vi "Get Status of Monkeys.vi"(8 "error in (no error)":errorcluster, 11 "Tamer in":refnum<class "Tamer.lvclass">) -> (0 "error out":errorcluster, 2 "Anything running?":bool, 3 "Tamer out":refnum<class "Tamer.lvclass">)   [LabVIEW 2020, in "Tamer.lvlib" / "Tamer.lvclass"]
doc: "Check if any Monkey is running"
uses:
  Tamer.lvclass
  Tamer.lvclass/Tamer.ctl
  Ancestor/Ancestor/Ancestor.lvclass/Ancestor.ctl
  Support VIs/Generate Error.vi
  FGV/Error Memory/Get Error Description.vi
  Support VIs/Get PC name.vi
  Ancestor/Ancestor/Read ID.vi
  Support VIs/Get Class Name.vi
  <vilib>/Utility/error.llb/Clear Errors.vi
  FGV/Error Memory/Error Memory Core.vi
  <vilib>/AdvancedString/Delimited String to 1D String Array.vi
  Support VIs/Circus Root Path.vi
  FGV/Error Memory/Error Crt Lvl checker.vi
  FGV/Error Memory/Error Memory Core.vi/40c8088d-b597-4017-91af-faa98e00292e.vi
  FGV/Error Memory/Error Memory Core.vi/d4a3ab98-063c-4e44-b43d-fbdcfe6c2be2.vi
  Is status ongoing - enum.vi
  Support VIs/Global Memory.vi
  <vilib>/Utility/LVClass/Get LV Class Name.vi
  Support VIs/Is in Packed Library.vi
  Support VIs/TALOS Root path.vi
  Support VIs/Read CSV worksheet.vi
  Support VIs/Global Constants.vi
  <vilib>/Utility/error.llb/General Error Handler.vi
  Support VIs/Error Log.vi
  Ancestor/Ancestor/Ancestor.lvclass
  <vilib>/Comparison/Equal/Equal Functor/Equal Functor.lvclass
  TALOS.lvlib
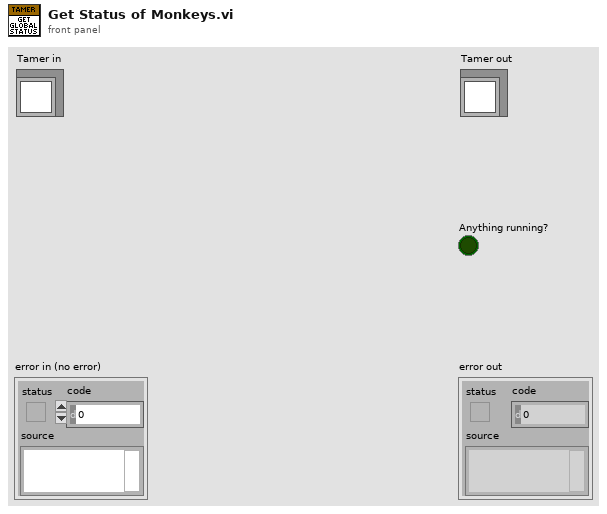
[diagram p1: front panel]
types:
  T1 = typedef "TALOS.lvlib/Run Utilities.lvlib/Monkey Status.ctl" = enum16{"Init", "Paused", "Ongoing", "Stopped", "Finished (no errors)", "Finished (with errors)"}
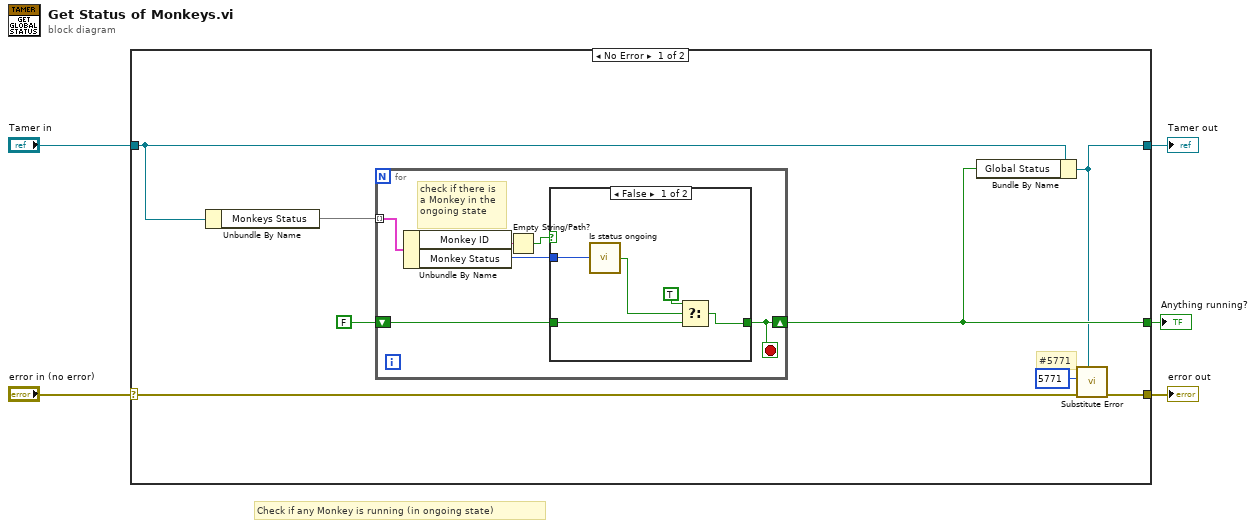
[diagram p0: block diagram]
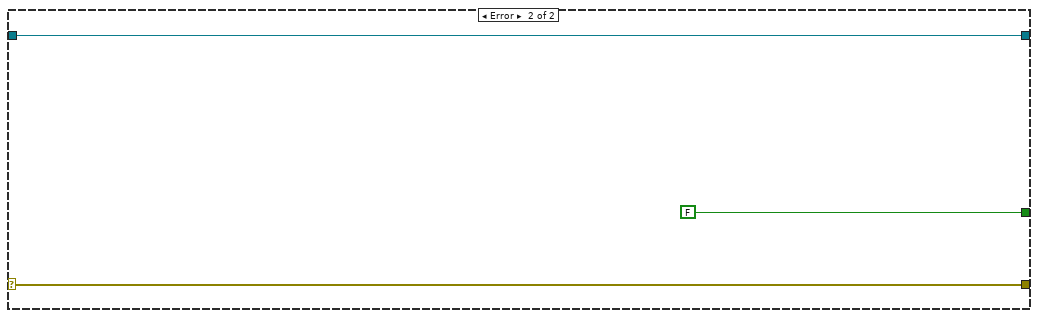
[diagram p3: hidden frame]
diagram:
  # "Check if any Monkey is running (in ongoing state)"
  n1 = case shown="No Error" "error in (no error)" {
    selector: "error in (no error)" -> [w6 w28]
    tunnel: [w13 w28] -> w4
    tunnel: [w10 w27] -> w2
    tunnel: "Tamer in" -> [w8 w27]
    tunnel: [w11 FALSE] -> w1
    frame No Error {
      # "#5771"
      n2 = Unbundle By Name(w8) -> ("Monkeys Status"=w9:map{string, T1})
      n3 = for {
        tunnel: w9 -> [w19] mode=indexing
        shift-right: [w17] -> w11
        shift-left: FALSE -> [w18]
        stop <- w17 stop-if-true
        # "check if there is a Monkey in the ongoing state"
        n4 = Unbundle By Name(w19) -> ("Monkey ID"=w15:string, "Monkey Status"=w14:T1)
        n5 = Empty String/Path?(string/path=w15) -> (empty?=w16:bool)
        n6 = case shown="False" w16 {
          tunnel: w14 -> [w22 _]
          tunnel: w18 -> [w24 w25]
          tunnel: [w23 w25] -> w17
          frame False {
            n7 = call-poly "Is status ongoing.vi"("Monkey Status"=w22) -> ("Monkey Running?"=w20:bool)
            n8 = Select(t=TRUE, s=w20, f=w24) -> (s? t:f=w23:bool)
          }
          frame True {
            # "Empty string, this is a patted value from converting 1D into 2D, ignore"
          }
        }
      }
      n9 = Bundle By Name(cluster=w8, "Global Status"=w11) -> (w10:refnum<class "Tamer.lvclass">)
      n10 = call "Substitute Error.vi"("LabVIEW Object"=w10, "error in (no error)"=w6, "Error Code"=5771) -> ("error out"=w13:errorcluster)  [unwired: 8 in]
    }
    frame Error {
    }
  }
  "error out" <- w4
  "Tamer out" <- w2
  "Anything running?" <- w1
